vi "model correction.vi"(8 "encoder count":dbl, 9 "stand position":dbl, 10 "encoder":dbl, 11 "virtual position":dbl) -> (1 "encoder position(Deg)":dbl, 2 "set position":dbl)   [LabVIEW 2019]
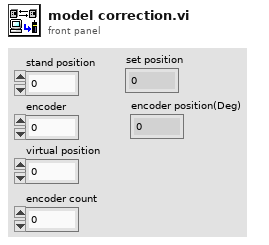
[diagram p1: front panel]
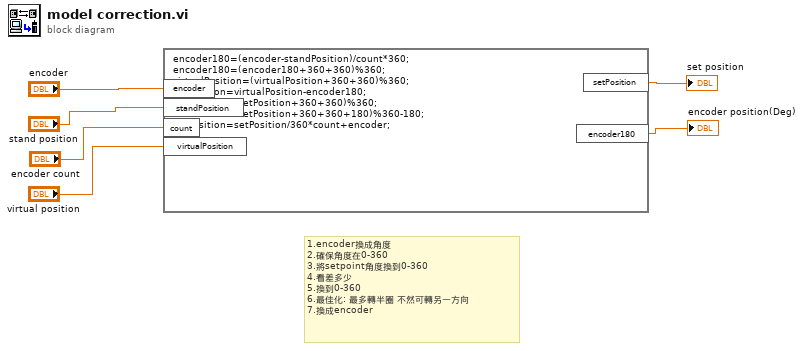
[diagram p0: block diagram]
diagram:
  # "1.encoder換成角度\n2.確保角度在0-360\n3.將setpoint角度換到0-360\n4.看差多少\n5.換到0-360\n6.最佳化: 最多轉半圈 不然可轉另一方向\n7.換成encoder"
  n1 = formula code="encoder180=(encoder-standPosition)/count*360;\nencoder180=(encoder180+360+360)%360;\nvirtualPosition=(virtualPosition+360+360)%360;\nsetPosition=virtualPosition-encoder180;\nsetPosition=(setPosition+360+360)%360;\nsetPosition=(setPosition+360+360+180)%360-180;\nsetPosition=setPosition/360*count+encoder;"("encoder"="encoder", "standPosition"="stand position", "count"="encoder count", "virtualPosition"="virtual position") -> ("setPosition"=→"set position":dbl, "encoder180"=→"encoder position(Deg)":dbl)
